vi "Write State to File.vi"(0 "Display State In":T1, 5 "tdms file":refnum<k34>, 7 "Lable.Text":string, 9 "Container State":T2, 11 "error in (no error)":errorcluster) -> (4 "Display State Out":T1, 6 "tdms file out":refnum<k34>, 15 "error out":errorcluster)   [LabVIEW 2015, in "Dynamic Device List.xctl"]
uses:
  Dynamic Device List.xctl
  <vilib>/_xctls/Container State.ctl
  Dynamic FP container.llb/Dynamic FP State.ctl
  Device/Device.lvclass
  Dynamic FP XControl/Name type and data.ctl
  Device/Device type.ctl
  Device/Read Name.vi
  Device/Read Controls Snapshot.vi
  <vilib>/_xctls/XControlSupport.lvlib
panel:
  # "Add Controls & Indicators that form the parameters of the method here. Hook them to the connector pane. Do not delete the controls & indicators that are already hooked to the connector pane.\n \nTo setup the parameters  for this method, right click on this item in the Project Tree & select \"Configure Method...\"."
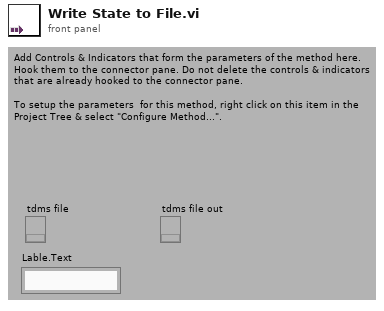
[diagram p1: front panel]
types:
  T1 = typedef "Dynamic Device List.xctl/Dynamic FP State.ctl" = cluster{"Complete device list":refnum<class "Device.lvclass">[], "Boolean test":bool, "Selected devices":u16[]}
  T2 = typedef "XControlSupport.lvlib/Container State.ctl" = cluster{"Indicator?":bool, "Run Mode?":bool, " Refnum":refnum<vi>}
  T3 = typedef "Name type and data.ctl" = cluster{"Front Panel Data":variant, "Device type":T4, "Name":string}
  T4 = typedef "Device type.ctl" = enum16{"NONE", "Neocera 21", "LakeShore 335", "LakeShore 340", "LkShr 340 chA&B", "LakeShore 370", "SRS 850", "SRS 830", "LR 700", "EG&G 5302", "EG&G 7260", "EG&G 7280", "AH 2500", "Keithley meter", "Keithley electrometer", "Keithley 182", "HP 5385", "HP 53181", "HP 53132", "ITC503", "IPS120", "Oxford Mercury IPS", "Oxford PS", "Test", "DC Facility Magnet", "Cryomagnetics PS", "Keithley 2400", "Keithley current source", "Cryo-Con 22C", "HP87NN", "HP4395A"}
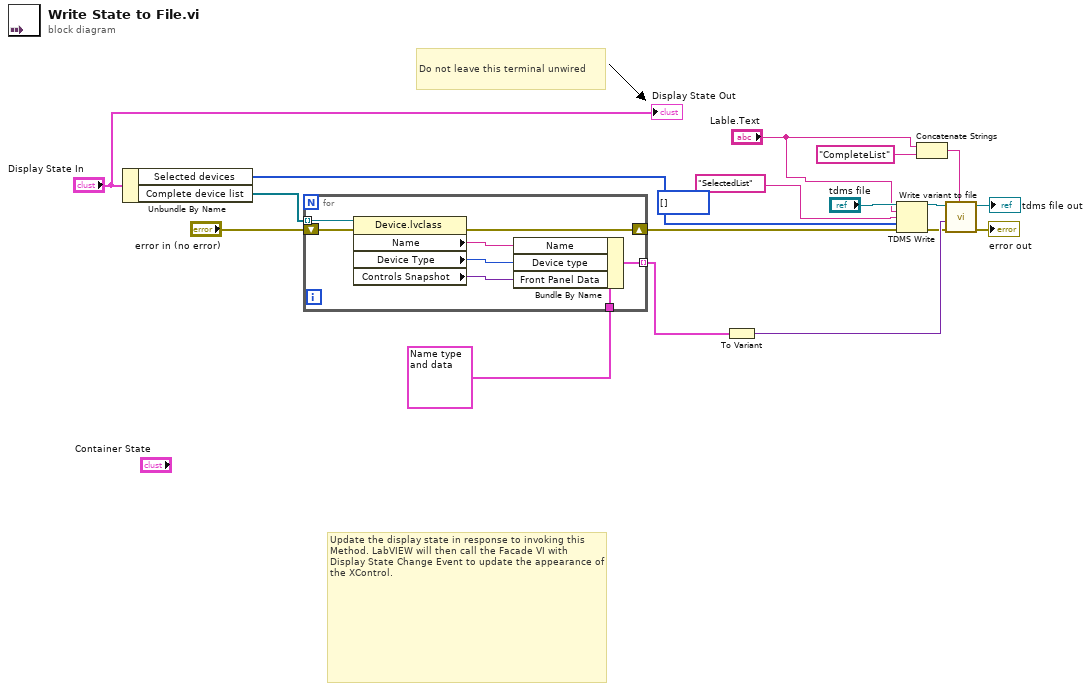
[diagram p0: block diagram]
diagram:
  (unwired) u16[] [] ("Selected devices")
  # "Do not leave this terminal unwired"
  # "Update the display state in response to invoking this Method. LabVIEW will then call the Facade VI with Display State Change Event to update the appearance of the XControl."
  n1 = Unbundle By Name("Display State In") -> ("Selected devices"=w3:u16[], "Complete device list"=w16:refnum<class "Device.lvclass">[])
  n2 = for {
    tunnel: w16 -> [w25] mode=indexing
    tunnel: [w23] -> w15 mode=indexing
    shift-right: [w20] -> w8
    shift-left: "error in (no error)" -> [w21]
    tunnel: T3 {"Front Panel Data"=variant, "Device type"=enum."NONE", "Name"=""} ("Name type and data") -> [w19]
    n3 = property class="Device.lvclass"(reference=w25, error in=w21) -> (error out=w20:errorcluster, "Name"=w22:string, "Device Type"=w18:T4, "Controls Snapshot"=w24:variant)  [unwired: 1 out]
    n4 = Bundle By Name(cluster=w19, "Name"=w22, "Device type"=w18, "Front Panel Data"=w24) -> (w23:T3)
  }
  n5 = To Variant(anything=w15) -> (Variant=w14:variant)
  n6 = TDMS Write(0:"tdms file", 5:"Lable.Text", 7:"SelectedList" ("string"), 9:w3, 11:w8) -> (4:w6:refnum<k34>, 15:w9:errorcluster)  [unwired: 1 in, 2 out]
  n7 = Concatenate Strings("Lable.Text", "CompleteList" ("string")) -> (w12:string)
  n8 = call "Write variant to file.vi"("error in (no error)"=w9, "variant"=w14, "Group name"=w12, "tdms file"=w6) -> ("error out"=→"error out":errorcluster, "tdms file out"=→"tdms file out":refnum<k34>)  [unwired: 6 in]
  "Display State Out" <- "Display State In"
